vi "Close.vi"(8 "error in (no error)":errorcluster, 11 "PacificPowerSource in":refnum<class "PacificPowerSource.lvclass">) -> (0 "error out":errorcluster, 3 "PacificPowerSource out":refnum<class "PacificPowerSource.lvclass">)   [LabVIEW 2018, in "AcPwrPlugins.lvlib" / "PacificPowerSource.lvclass"]
doc: "This VI closes the reference to the instrument."
uses:
  PacificPowerSource.lvclass
  <instrlib>/Pacific Power UPC Series/Pacific Power UPC Series.lvlib
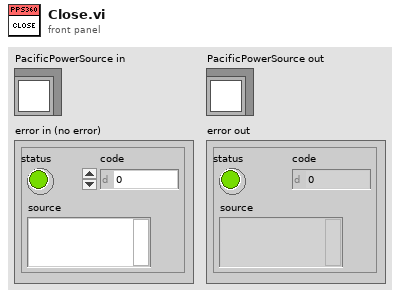
[diagram p1: front panel]
types:
  T1 = typedef "AcPwrPlugins.lvlib/PacificPowerSource.lvclass/Device(s)Settings.ctl" = cluster{"MeasName":string, "Modules":cluster{"Handle":string, "Connected":bool, "Clear Device (F)":bool, "btnIdQuery":bool, "btnReset":bool, "Program #":cluster{"Phase B (Degrees)":i32, "Waveform A (1: Sine)":i32, "Voltage Level (Va)":dbl, "Program Number (0)":i32, "Voltage Level (Vb) ":dbl, "Form (3: Three)":u16, "Coupling  (0: Direct)":u16, "Frequency (45Hz)":dbl, "Current Limit (40A)":dbl, "Phase C (Degrees)":i32, "Voltage Level (Vc)":dbl, "Waveform B (1: Sine)":i32, "Waveform C (1: Sine)":i32}[], "Impedance Parameters (off, 0.00)":cluster{"State":bool, "Impedance":dbl}, "Transient Execution (F)":bool, "OutputEnabled":bool, "Source Range":cluster{"Frequency Minimum (45 Hz)":dbl, "Frequency Maximum (1200 Hz)":dbl, "Voltage Maximum (V)":dbl, "Voltage Minimum (V)":dbl, "Range Control (0: Auto)":u16, "Initial Voltage (0V)":dbl, "Frequency Range (600Hz)":u16}, "Port Type":enum16{"GPIB", "Serial"}}[]}
  T2 = typedef "AcPwrPlugins.lvlib/PacificPowerSource.lvclass/Measurements.ctl" = cluster{"Handle":string, "Name":string, "Enabled ":bool, "Measurement Value":dbl, "Channel Name":enum16{"A", "B", "C"}, "Measurement Type ":T3}[]
  T3 = typedef "AcPwrPlugins.lvlib/PacificPowerSource.lvclass/MeasurementType.ctl" = enum16{"Voltage RMS L-N", "Voltage RMS L-L", "Frequency", "Current RMS", "Current Peak", "Crest Factor", "Power Factor", "Power VA", "Real Power"}
  T4 = typedef "AcPwrPlugins.lvlib/PacificPowerSource.lvclass/Modules.ctl" = cluster{"Handle":string, "Connected":bool, "Clear Device (F)":bool, "btnIdQuery":bool, "btnReset":bool, "Program #":cluster{"Phase B (Degrees)":i32, "Waveform A (1: Sine)":i32, "Voltage Level (Va)":dbl, "Program Number (0)":i32, "Voltage Level (Vb) ":dbl, "Form (3: Three)":u16, "Coupling  (0: Direct)":u16, "Frequency (45Hz)":dbl, "Current Limit (40A)":dbl, "Phase C (Degrees)":i32, "Voltage Level (Vc)":dbl, "Waveform B (1: Sine)":i32, "Waveform C (1: Sine)":i32}[], "Impedance Parameters (off, 0.00)":cluster{"State":bool, "Impedance":dbl}, "Transient Execution (F)":bool, "OutputEnabled":bool, "Source Range":cluster{"Frequency Minimum (45 Hz)":dbl, "Frequency Maximum (1200 Hz)":dbl, "Voltage Maximum (V)":dbl, "Voltage Minimum (V)":dbl, "Range Control (0: Auto)":u16, "Initial Voltage (0V)":u16, "Frequency Range (600Hz)":u16}, "Port Type":enum16{"GPIB", "Serial"}}[]
  T5 = cluster{"Handle":string, "Connected":bool, "Clear Device (F)":bool, "btnIdQuery":bool, "btnReset":bool, "Program #":cluster{"Phase B (Degrees)":i32, "Waveform A (1: Sine)":i32, "Voltage Level (Va)":dbl, "Program Number (0)":i32, "Voltage Level (Vb) ":dbl, "Form (3: Three)":u16, "Coupling  (0: Direct)":u16, "Frequency (45Hz)":dbl, "Current Limit (40A)":dbl, "Phase C (Degrees)":i32, "Voltage Level (Vc)":dbl, "Waveform B (1: Sine)":i32, "Waveform C (1: Sine)":i32}[], "Impedance Parameters (off, 0.00)":cluster{"State":bool, "Impedance":dbl}, "Transient Execution (F)":bool, "OutputEnabled":bool, "Source Range":cluster{"Frequency Minimum (45 Hz)":dbl, "Frequency Maximum (1200 Hz)":dbl, "Voltage Maximum (V)":dbl, "Voltage Minimum (V)":dbl, "Range Control (0: Auto)":u16, "Initial Voltage (0V)":u16, "Frequency Range (600Hz)":u16}, "Port Type":enum16{"GPIB", "Serial"}}
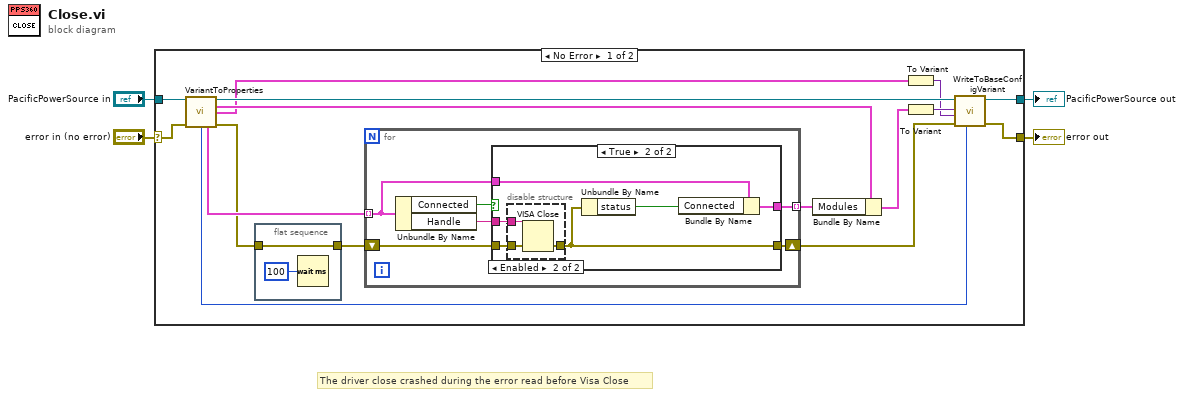
[diagram p0: block diagram]
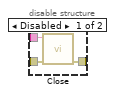
[diagram p3: hidden frame]
diagram:
  # "The driver close crashed during the error read before Visa Close"
  n1 = case shown="No Error" "error in (no error)" {
    selector: "error in (no error)" -> [w18 w44]
    tunnel: [w10 w44] -> w4
    tunnel: [w14 w43] -> w3
    tunnel: "PacificPowerSource in" -> [w19 w43]
    frame No Error {
      n2 = call "VariantToProperties.vi"("PacificPowerSource in"=w19, "error in (no error)"=w18) -> ("PacificPowerSource out"=w15:refnum<class "PacificPowerSource.lvclass">, "Device(s)Settings"=w16:T1, "Measurements"=w7:T2, "Measurement Refresh Time (ms)"=w9:u32, "Modules"=w17:T4, "error out"=w5:errorcluster)  [unwired: 7 in, 1 out]
      n3 = flat-sequence {
        tunnel: w5 -> [w21]
        tunnel: [w21] -> w6
        frame #0 {
          n4 = Wait (ms)(milliseconds to wait=u32 100) -> ()  [unwired: 1 out]
        }
      }
      n5 = for {
        shift-right: [w27] -> w13
        shift-left: w6 -> [w28]
        tunnel: w17 -> [w24] mode=indexing
        tunnel: [w23] -> w20 mode=indexing
        n6 = Unbundle By Name(w24) -> ("Connected"=w25:bool, "Handle"=w26:string)
        n7 = case shown="True" w25 {
          tunnel: w28 -> [w30 w36]
          tunnel: [w30 w32] -> w27
          tunnel: w26 -> [_ w35]
          tunnel: w24 -> [w29 w34]
          tunnel: [w29 w33] -> w23
          frame False {
          }
          frame True {
            n8 = disable-structure shown="Enabled" {
              disable-tunnel: w36 -> [w39 w42]
              disable-tunnel: w35 -> [w38 w41]
              disable-tunnel: [w37 w40] -> w32
              frame Disabled {
                n9 = call <instrlib>:"Close.vi"("error in (no error)"=w39, "VISA resource name"=w38) -> ("error out"=w37:errorcluster)  [unwired: 9 in]
              }
              frame Enabled {
                n10 = VISA Close(VISA resource name=w41, error in (no error)=w42) -> (error out=w40:errorcluster)
              }
            }
            n11 = Unbundle By Name(w32) -> ("status"=w31:bool)
            n12 = Bundle By Name(cluster=w34, "Connected"=w31) -> (w33:T5)
          }
        }
      }
      n13 = Bundle By Name(cluster=w16, "Modules"=w20) -> (w11:T1)
      n14 = To Variant(anything=w7) -> (Variant=w8:variant)
      n15 = To Variant(anything=w11) -> (Variant=w12:variant)
      n16 = call "WriteToBaseConfigVariant.vi"("Measurement Refresh Time (ms)"=w9, "error in (no error)"=w13, "Meas"=w8, "Config"=w12, "PacificPowerSource in"=w15) -> ("error out"=w10:errorcluster, "PacificPowerSource out"=w14:refnum<class "PacificPowerSource.lvclass">)  [unwired: 5 in]
    }
    frame Error {
    }
  }
  "error out" <- w4
  "PacificPowerSource out" <- w3
